vi "Keithley 24XX Sweep and Acquire Measurements.vi"() -> ()   [LabVIEW 2017]
doc: "Configures a sweep and takes voltage and current readings at each point."
uses:
  <instrlib>/Keithley 24XX/Public/Data/Read (Multiple Points).vi
  <instrlib>/Keithley 24XX/Keithley 24XX.lvlib
panel:
  in  "Source Mode  (0: Voltage)":u16(ring) items=["Voltage", "Current"]
  in  "Serial Configuration":T1={"Baud Rate"=9600, "Parity"=0, "Data Bits"=8, "Stop Bits"=10, "Flow Control"=0} {"Flow Control" items=["None", "XON/XOFF", "RTS/CTS", "XON/XOFF & RTS/CTS", "DTR/DSR", "XON/XOFF & DTR/DSR"]; "Stop Bits" items=["1.0"=10, "1.5"=15, "2.0"=20]; "Data Bits" items=["7"=7, "8"=8]; "Parity" items=["None", "Odd", "Even", "Mark", "Space"]; "Baud Rate" items=["300"=300, "600"=600, "1200"=1200, "2400"=2400, "4800"=4800, "9600"=9600, "19200"=19200]}
  in  "VISA resource name":refnum<visa-resource-name>
  out "Waveform Graph":sgl[][](graph)
  in  "Timeout (10000 ms)":i32=10000 format="%#.6g"
  in  "Maximum Amplitude (2)":dbl=2.0
  in  "Minimum Amplitude (1)":dbl=1.0
  in  "Number of Points (5)":u32=5
  in  "Compliance  Level (0.1)":dbl=0.1
  # "(c) 2006 - 2015 National Instruments.  ALL RIGHTS RESERVED."
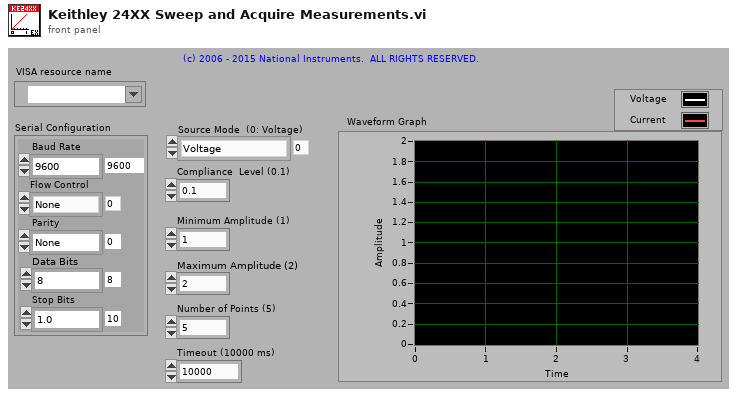
[diagram p1: front panel]
types:
  T1 = cluster{"Baud Rate":u32, "Parity":u16, "Data Bits":u16, "Stop Bits":u16, "Flow Control":u16}
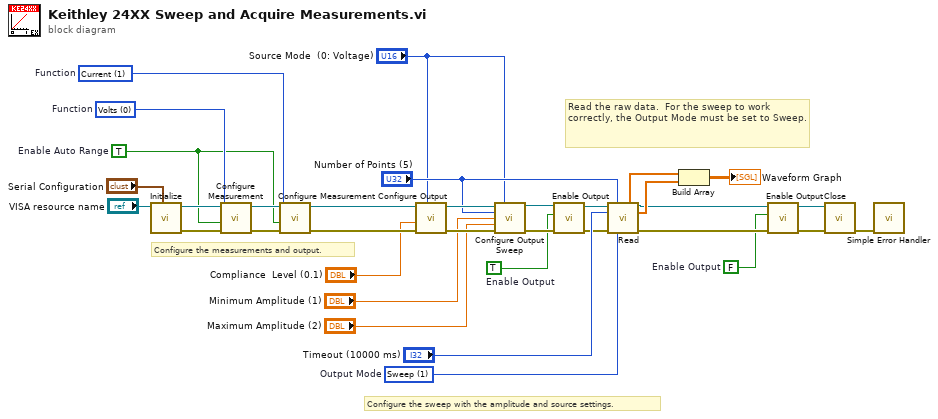
[diagram p0: block diagram]
diagram:
  w2 = TRUE  # Enable Output
  w3 = TRUE  # Enable Auto Range
  w4 = u16 1 items=["Volts", "Current", "Resistance"]  # Function
  w5 = u16 0 items=["Volts", "Current", "Resistance"]  # Function
  w11 = FALSE  # Enable Output
  w17 = u16 1 items=["Fixed", "Sweep", "List"]  # Output Mode
  # "Read the raw data.  For the sweep to work correctly, the Output Mode must be set to Sweep."
  # "Configure the sweep with the amplitude and source settings."
  # "Configure the measurements and output."
  n1 = call <instrlib>:"Initialize.vi"("Serial Configuration"="Serial Configuration", "VISA resource name"="VISA resource name") -> ("error out"=w33:errorcluster, "VISA resource name out"=w34:refnum<visa-resource-name>)  [unwired: 8 in]
  n2 = call <instrlib>:"Configure Measurement.vi"("error in (no error)"=w33, "Enable Auto Range (T:Enable)"=w3, "Function (0: Volts)"=w5, "VISA resource name"=w34) -> ("error out"=w32:errorcluster, "VISA resource name out"=w31:refnum<visa-resource-name>)  [unwired: 6 in]
  n3 = call <instrlib>:"Configure Measurement.vi"("error in (no error)"=w32, "Enable Auto Range (T:Enable)"=w3, "Function (0: Volts)"=w4, "VISA resource name"=w31) -> ("error out"=w29:errorcluster, "VISA resource name out"=w30:refnum<visa-resource-name>)  [unwired: 6 in]
  n4 = call <instrlib>:"Configure Output.vi"("Source Mode  (0: Voltage)"="Source Mode  (0: Voltage)", "error in (no error)"=w29, "Compliance  Level (0.1)"="Compliance  Level (0.1)", "VISA resource name"=w30) -> ("error out"=w28:errorcluster, "VISA resource name out"=w27:refnum<visa-resource-name>)  [unwired: 6 in]
  n5 = call <instrlib>:"Configure Output Sweep.vi"("VISA resource name"=w27, "Source Mode  (0: Voltage)"="Source Mode  (0: Voltage)", "Number of Points (5)"="Number of Points (5)", "Minimum Amplitude (1)"="Minimum Amplitude (1)", "Maximum Amplitude (2)"="Maximum Amplitude (2)", "error in (no error)"=w28) -> ("VISA resource name out"=w8:refnum<visa-resource-name>, "error out"=w7:errorcluster)  [unwired: 8 in]
  n6 = call <instrlib>:"Enable Output.vi"("error in (no error)"=w7, "Enable Output (T: Enable)"=w2, "VISA resource name"=w8) -> ("error out"=w10:errorcluster, "VISA resource name out"=w9:refnum<visa-resource-name>)  [unwired: 7 in]
  n7 = call-poly <instrlib>:"Read.vi"("VISA resource name"=w9, "Sample Count (1)"="Number of Points (5)", "Timeout (10000 ms)"="Timeout (10000 ms)", "error in (no error)"=w10, "Output Mode (0: Fixed)"=w17) -> ("Voltage"=w22:sgl[], "VISA resource name out"=w12:refnum<visa-resource-name>, "Current"=w21:sgl[], "error out"=w13:errorcluster)  [unwired: 4 in, 3 out]
  n8 = Build Array(w22, w21) -> (→"Waveform Graph":sgl[][])
  n9 = call <instrlib>:"Enable Output.vi"("error in (no error)"=w13, "Enable Output (T: Enable)"=w11, "VISA resource name"=w12) -> ("error out"=w14:errorcluster, "VISA resource name out"=w15:refnum<visa-resource-name>)  [unwired: 7 in]
  n10 = call <instrlib>:"Close.vi"("error in (no error)"=w14, "VISA resource name"=w15) -> ("error out"=w16:errorcluster)  [unwired: 9 in]
  n11 = call <vilib>:"Simple Error Handler.vi"("error in (no error)"=w16) -> ()  [unwired: 4 in, 5 out]
